vi "UT_EField_DAQ_AnalogIO.get outputs.vi"(0 "i ref in":refnum<vi>, 3 "Timeout":i32=10000, 5 "error in":errorcluster caption="Fehler (Eingang, kein Fehler)") -> (7 "scale_factor":dbl, 9 "physical_channels":string[](array[string]), 11 "virtual_channels":string[](array[string]), 13 "range":cluster{"min":dbl, "max":dbl}[](array[cluster]), 14 "i ref out":refnum<vi>, 16 "channel_index":i32[](array[numeric]), 19 "error out":errorcluster caption="Fehler (Ausgang)")   [LabVIEW 2014, in "UT_EField_DAQ_AnalogIO.lvlib"]
doc: "Contact: Falk Ziegler, eMail: info@lab-coding.de"
uses:
  UT_EField_DAQ_AnalogIO.lvlib
  <vilib>/regexp/Match Regular Expression.xnode
  CS_Core/BaseProcess/BaseProcess.lvlib
panel:
  in  "port_data_type":T1
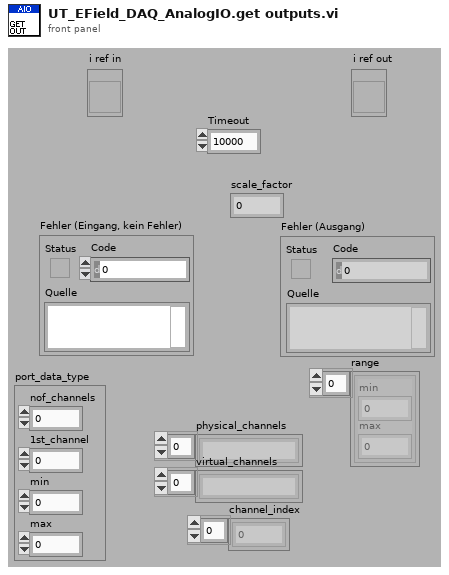
[diagram p1: front panel]
types:
  T1 = cluster{"nof_channels":i32, "1st_channel":i32, "min":dbl, "max":dbl}
  T2 = cluster{"nof_channels":i32, "1st_channel":i32, "min":dbl, "max":dbl}[]
  T3 = typedef "BaseProcess.lvlib/BaseProcess.i attribute.ctl" = cluster{"EventStatus":string, "EventError":i32, "PresetEvtWatchD":i32, "PresetPdcWatchD":i32, "EventTimeout":i32, "PeriodicInterval":i32, "Interface":string[], "Address":string[], "Special":string[], "PeriodicError":i32, "PeriodicStatus":string, "SuperProc":string, "Descriptors":T4[], "CaseRef":refnum<vi>, "PdcRef":refnum<vi>, "Thread Ref":refnum<vi>, "eventErrorID":i32, "eventStatusID":i32, "periodicErrorID":i32, "periodicStatusID":i32, "pdcCtrID":i32}
  T4 = typedef "BaseProcess.lvlib/BaseProcess.descriptor definition.ctl" = cluster{"selector":string, "descriptor":T5}
  T5 = typedef "BaseProcess.lvlib/BaseProcess.descriptor string definition.ctl" = string
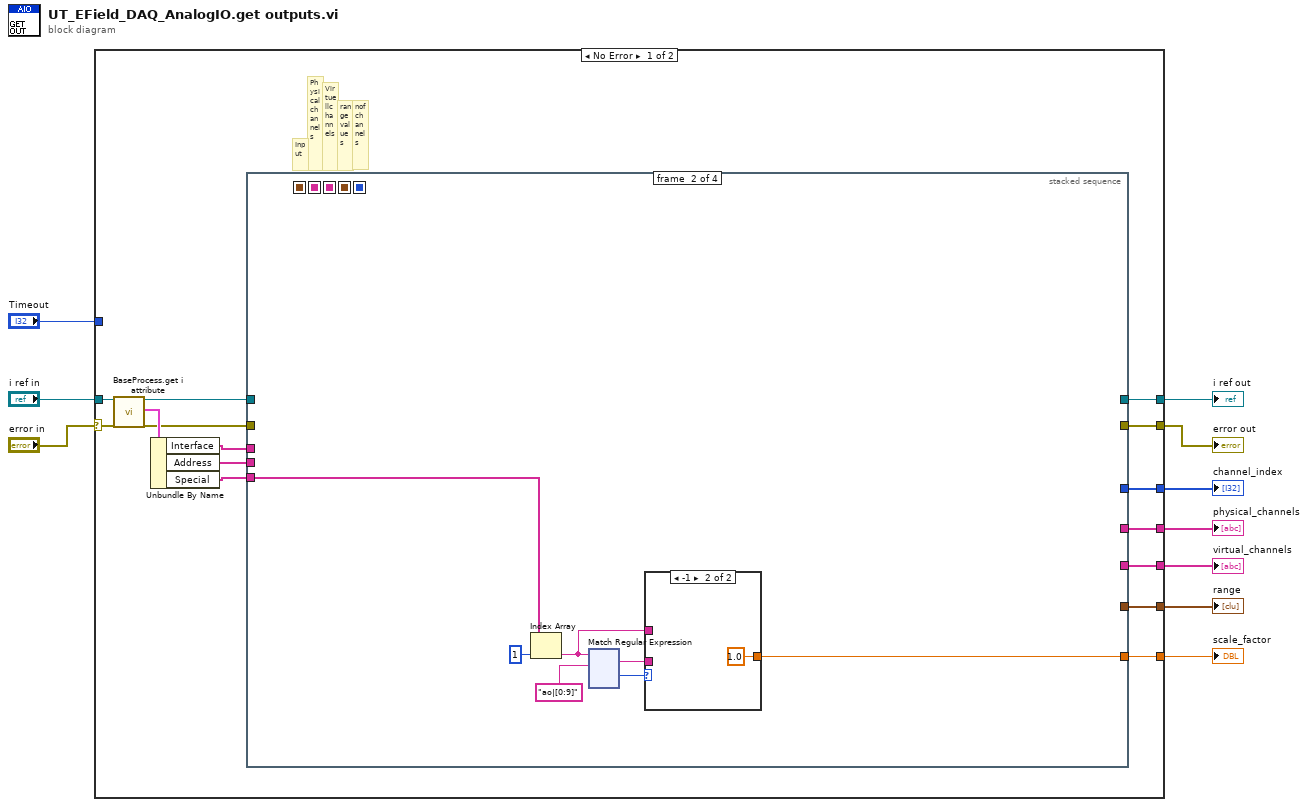
[diagram p0: block diagram]
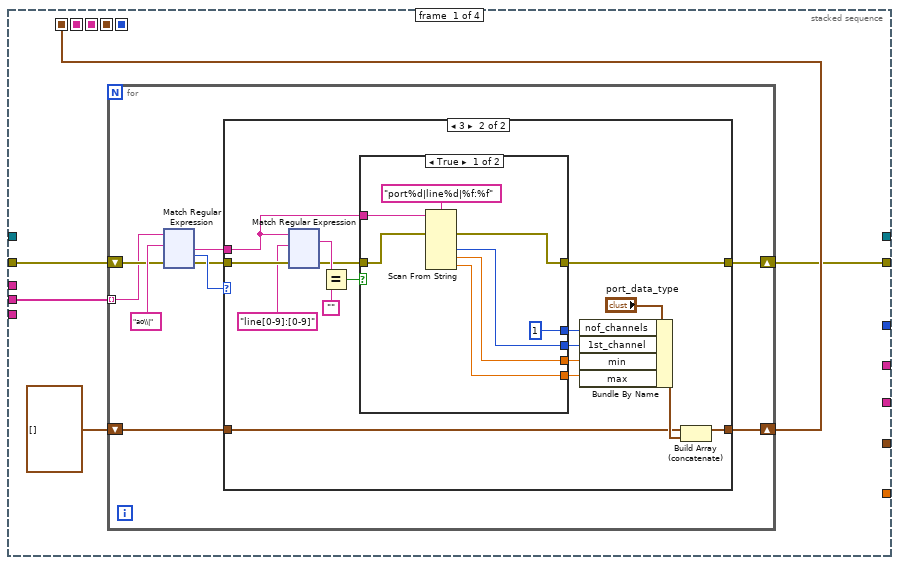
[diagram p2: hidden frame]
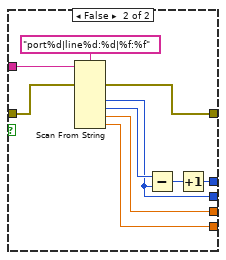
[diagram p4: hidden frame]
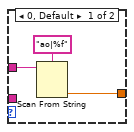
[diagram p5: hidden frame]
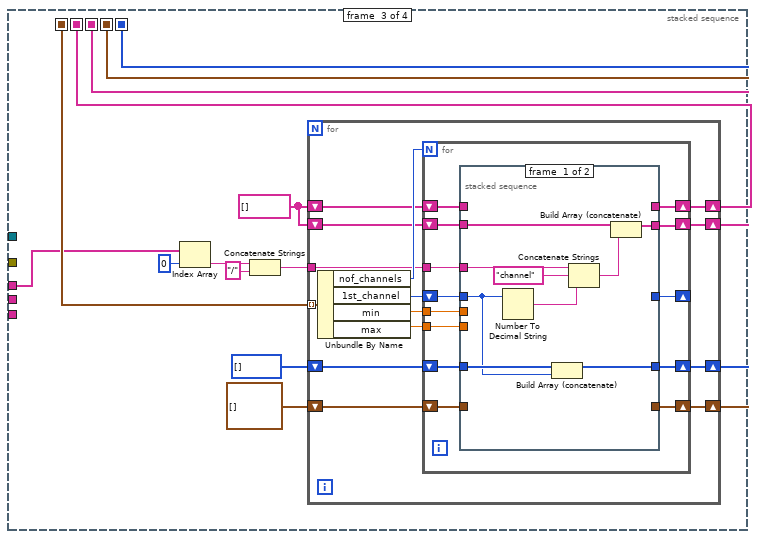
[diagram p6: hidden frame]
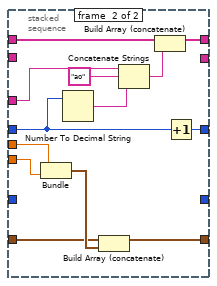
[diagram p7: hidden frame]
diagram:
  n1 = case shown="No Error" "error in" {
    selector: "error in" -> [w24 w488]
    tunnel: "i ref in" -> [w25 w487]
    tunnel: [w18 w488] -> w8
    tunnel: [w19 w487] -> w7
    tunnel: "Timeout" -> [_ _]
    tunnel: [w16 _] -> w5
    tunnel: [w15 _] -> w4
    tunnel: [w17 _] -> w2
    tunnel: [w14 _] -> w3
    tunnel: [w12 _] -> w1
    frame No Error {
      # "range values"
      # "nofchannels"
      # "Virtuellchannels"
      # "Physicalchannels"
      # "Input"
      n2 = call "BaseProcess.get i attribute.vi"("i ref in"=w25, "error in (no error)"=w24) -> ("i ref out"=w22:refnum<vi>, "i attribute"=w23:T3, "error out"=w21:errorcluster)  [unwired: 15 in]
      n3 = Unbundle By Name(w23) -> ("Interface"=w13:string[], "Address"=w20:string[], "Special"=w11:string[])
      n4 = stacked-sequence {
        seq-local: [w27 _ _ _] -> [_ _ w432 _]
        seq-local: [_ _ w429 _] -> [_ _ _ w486]
        seq-local: [_ _ w428 _] -> [_ _ _ w485]
        seq-local: [_ _ w427 _] -> [_ _ _ w482]
        seq-local: [_ _ w425 _] -> [_ _ _ w484]
        tunnel: w20 -> [w30 _ _ _]
        tunnel: [_ _ _ w486] -> w16
        tunnel: [_ _ _ w485] -> w15
        tunnel: [_ _ _ w482] -> w17
        tunnel: [_ _ _ w484] -> w14
        tunnel: w21 -> [w29 _ _ _]
        tunnel: w22 -> [_ _ _ w483]
        tunnel: [_ _ _ w483] -> w19
        tunnel: [w26 _ _ _] -> w18
        tunnel: w13 -> [_ _ w422 _]
        tunnel: [_ w300 _ _] -> w12
        tunnel: w11 -> [_ w299 _ _]
        frame #0 {
          n5 = for {
            shift-right: [w35] -> w26
            shift-left: w29 -> [w34]
            tunnel: w30 -> [w33] mode=indexing
            shift-right: [w32] -> w27
            shift-left: T2 [] -> [w31]
            n6 = xnode "Match Regular Expression"("input string"=w33, "regular expression"="ao\\|", "error in"=w34) -> ("after match"=w37:string, "offset past match"=w38:i32, "error out"=w36:errorcluster)  [unwired: 3 in, 2 out]
            n7 = case shown="3" w38 {
              tunnel: w37 -> [_ w52]
              tunnel: w36 -> [w41 w57]
              tunnel: [w41 w50] -> w35
              tunnel: [w40 w43] -> w32
              tunnel: w31 -> [w40 w42]
              frame 0, Default {
              }
              frame 3 {
                n8 = xnode "Match Regular Expression"("input string"=w52, "regular expression"="line[0-9]:[0-9]", "error in"=w57) -> ("whole match"=w55:string, "error out"=w51:errorcluster)  [unwired: 3 in, 3 out]
                n9 = Equal?(x=w55, y="") -> (x = y?=w54:bool)
                n10 = case shown="True" w54 {
                  tunnel: w52 -> [w65 w75]
                  tunnel: w51 -> [w63 w73]
                  tunnel: [w62 w72] -> w50
                  tunnel: [1 w66] -> w48
                  tunnel: [w59 w68] -> w47
                  tunnel: [w61 w70] -> w46
                  tunnel: [w60 w71] -> w45
                  frame True {
                    n11 = Scan From String(format string="port%d|line%d|%f:%f", input string=w65, error in=w63) -> (error out=w62:errorcluster, output 2=w59:i32, output 3=w61:dbl, output 4=w60:dbl)  [unwired: 6 in, 2 out]
                  }
                  frame False {
                    n12 = Scan From String(format string="port%d|line%d:%d|%f:%f", input string=w75, error in=w73) -> (error out=w72:errorcluster, output 2=w68:i32, output 3=w69:i32, output 4=w70:dbl, output 5=w71:dbl)  [unwired: 7 in, 2 out]
                    n13 = Subtract(x=w69, y=w68) -> (x-y=w67:i32)
                    n14 = Increment(x=w67) -> (x+1=w66:i32)
                  }
                }
                n15 = Bundle By Name(cluster="port_data_type", "nof_channels"=w48, "1st_channel"=w47, "min"=w46, "max"=w45) -> (w44:T1)
                n16 = Build Array (concatenate)(w42, w44) -> (w43:T2)
              }
            }
          }
        }
        frame #1 {
          n17 = Index Array(array=w299, index=1) -> (element=w301:string)
          n18 = xnode "Match Regular Expression"("input string"=w301, "regular expression"="ao|[0:9]") -> ("whole match"=w298:string, "offset past match"=w302:i32)  [unwired: 4 in, 3 out]
          n19 = case shown="-1" w302 {
            tunnel: w301 -> [w307 _]
            tunnel: [w305 1.0] -> w300
            tunnel: w298 -> [_ _]
            frame 0, Default {
              n20 = Scan From String(format string="ao|%f", input string=w307) -> (output 1=w305:dbl)  [unwired: 3 in, 3 out]
            }
            frame -1 {
            }
          }
        }
        frame #2 {
          w430 = string[] []
          n21 = Index Array(array=w422, index=0) -> (element=w420:string)
          n22 = Concatenate Strings(w420, "/" ("String")) -> (w423:string)
          n23 = for {
            tunnel: w432 -> [w446] mode=indexing
            shift-right: [w440] -> w428
            shift-left: w430 -> [w443]
            shift-right: [w442] -> w427
            shift-left: i32[] [] -> [w444]
            shift-right: [w438] -> w429
            shift-left: w430 -> [w439]
            shift-right: [w435] -> w425
            shift-left: cluster{"min":dbl, "max":dbl}[] [] -> [w434]
            tunnel: w423 -> [w433]
            n24 = Unbundle By Name(w446) -> ("nof_channels"=w445:i32, "1st_channel"=w441:i32, "min"=w437:dbl, "max"=w436:dbl)
            n25 = for {
              N: w445 -> [_]
              shift-right: [w457] -> w440
              shift-left: w443 -> [w456]
              shift-right: [w458] -> w442
              shift-left: w444 -> [w459]
              shift-right: [w453] -> _
              shift-left: w441 -> [w455]
              shift-right: [w452] -> w438
              shift-left: w439 -> [w454]
              tunnel: w437 -> [w451]
              tunnel: w436 -> [w450]
              shift-right: [w449] -> w435
              shift-left: w434 -> [w448]
              tunnel: w433 -> [w447]
              n26 = stacked-sequence {
                tunnel: w459 -> [w462 _]
                tunnel: [w461 _] -> w458
                tunnel: [w466 _] -> w457
                tunnel: w456 -> [w465 _]
                tunnel: w455 -> [w460 w479]
                tunnel: w454 -> [_ w477]
                tunnel: [_ w480] -> w453
                tunnel: [_ w476] -> w452
                tunnel: w451 -> [_ w473]
                tunnel: w450 -> [_ w474]
                tunnel: [_ w471] -> w449
                tunnel: w448 -> [_ w470]
                tunnel: w447 -> [w463 w469]
                frame #0 {
                  n27 = Number To Decimal String(number=w460) -> (decimal integer string=w467:string)  [unwired: 1 in]
                  n28 = Build Array (concatenate)(w462, w460) -> (w461:i32[])
                  n29 = Concatenate Strings(w463, "channel" ("String"), w467) -> (w464:string)
                  n30 = Build Array (concatenate)(w465, w464) -> (w466:string[])
                }
                frame #1 {
                  n31 = Bundle("min"=w473, "max"=w474) -> (w472:cluster{"min":dbl, "max":dbl})  [unwired: 1 in]
                  n32 = Number To Decimal String(number=w479) -> (decimal integer string=w478:string)  [unwired: 1 in]
                  n33 = Build Array (concatenate)(w470, w472) -> (w471:cluster{"min":dbl, "max":dbl}[])
                  n34 = Concatenate Strings(w469, "ao" ("String"), w478) -> (w475:string)
                  n35 = Build Array (concatenate)(w477, w475) -> (w476:string[])
                  n36 = Increment(x=w479) -> (x+1=w480:i32)
                }
              }
            }
          }
        }
        frame #3 {
        }
      }
    }
    frame Error {
    }
  }
  "error out" <- w8
  "i ref out" <- w7
  "physical_channels" <- w5
  "virtual_channels" <- w4
  "range" <- w3
  "channel_index" <- w2
  "scale_factor" <- w1
